vi "MANUALGCODE.vi"(8 "error in (no error)":errorcluster, 9 "PARA":cluster{"STEP":i16, "FEEDRATE":dbl} {"STEP" min=0 max=90 step=2 format="%-1.0f"}, 10 "STATE\nSTAT":enum16{"X-", "X+", "Y-", "Y+", "Z-", "Z+"}(ring), 11 "QUEUE IN":refnum<queue>) -> (0 "error out":errorcluster)   [LabVIEW 2017]
panel:
  out "concatenated string":string
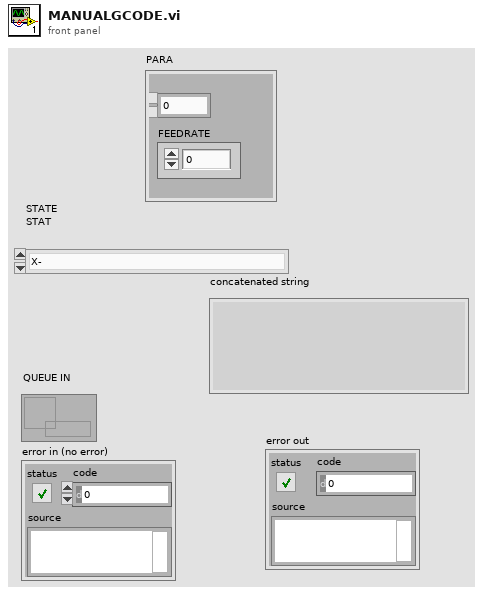
[diagram p1: front panel]
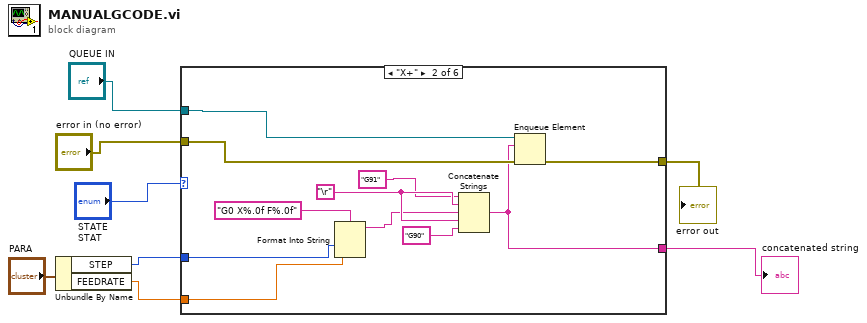
[diagram p0: block diagram]
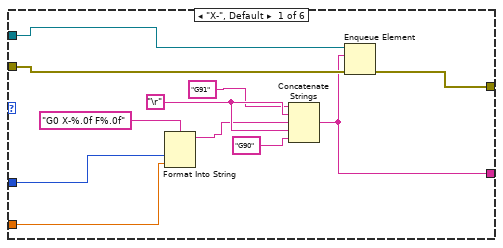
[diagram p2: hidden frame]
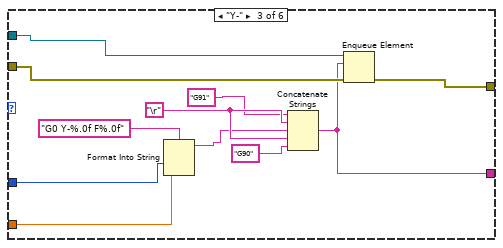
[diagram p3: hidden frame]
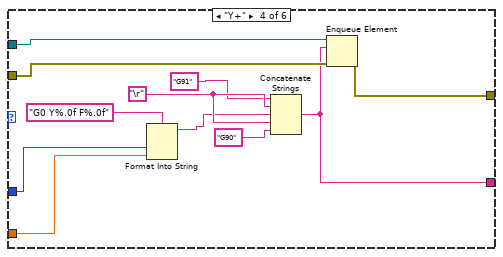
[diagram p4: hidden frame]
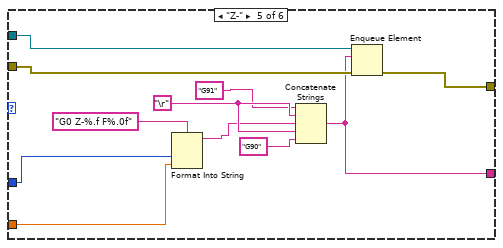
[diagram p5: hidden frame]
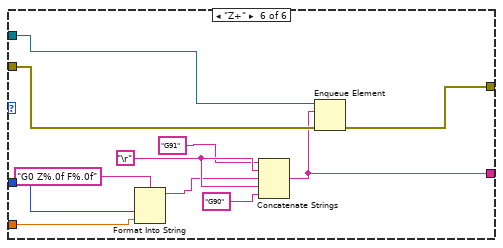
[diagram p6: hidden frame]
diagram:
  n1 = Unbundle By Name("PARA") -> ("STEP"=w1:i16, "FEEDRATE"=w2:dbl)
  n2 = case shown="\"X+\"" "STATE\nSTAT" {
    tunnel: "QUEUE IN" -> [w13 w27 w35 w47 w58 w68]
    tunnel: "error in (no error)" -> [w12 w26 w34 w46 w57 w67]
    tunnel: [w14 w25 w36 w45 w56 w69] -> w5
    tunnel: w2 -> [w10 w20 w31 w43 w54 w65]
    tunnel: [w11 w22 w33 w44 w55 w66] -> w4
    tunnel: w1 -> [w9 w21 w32 w42 w53 w64]
    frame "X-", Default {
      w19 = "\r"
      n3 = Format Into String(format string="G0 X-%.0f F%.0f", w9, w10) -> (resulting string=w15:string)  [unwired: 2 in, 1 out]
      n4 = Concatenate Strings("G91" ("string"), w19, w15, w19, "G90" ("string")) -> (w11:string)
      n5 = Enqueue Element(queue=w13, element=w11, error in (no error)=w12) -> (error out=w14:errorcluster)  [unwired: 1 in, 2 out]
    }
    frame "X+" {
      w30 = "\r"
      n6 = Format Into String(format string="G0 X%.0f F%.0f", w21, w20) -> (resulting string=w23:string)  [unwired: 2 in, 1 out]
      n7 = Concatenate Strings("G91" ("string"), w30, w23, w30, "G90" ("string")) -> (w22:string)
      n8 = Enqueue Element(queue=w27, element=w22, error in (no error)=w26) -> (error out=w25:errorcluster)  [unwired: 1 in, 2 out]
    }
    frame "Y-" {
      w41 = "\r"
      n9 = Format Into String(format string="G0 Y-%.0f F%.0f", w32, w31) -> (resulting string=w37:string)  [unwired: 2 in, 1 out]
      n10 = Concatenate Strings("G91" ("string"), w41, w37, w41, "G90" ("string")) -> (w33:string)
      n11 = Enqueue Element(queue=w35, element=w33, error in (no error)=w34) -> (error out=w36:errorcluster)  [unwired: 1 in, 2 out]
    }
    frame "Y+" {
      w52 = "\r"
      n12 = Format Into String(format string="G0 Y%.0f F%.0f", w42, w43) -> (resulting string=w48:string)  [unwired: 2 in, 1 out]
      n13 = Concatenate Strings("G91" ("string"), w52, w48, w52, "G90" ("string")) -> (w44:string)
      n14 = Enqueue Element(queue=w47, element=w44, error in (no error)=w46) -> (error out=w45:errorcluster)  [unwired: 1 in, 2 out]
    }
    frame "Z-" {
      w63 = "\r"
      n15 = Format Into String(format string="G0 Z-%.f F%.0f", w53, w54) -> (resulting string=w59:string)  [unwired: 2 in, 1 out]
      n16 = Concatenate Strings("G91" ("string"), w63, w59, w63, "G90" ("string")) -> (w55:string)
      n17 = Enqueue Element(queue=w58, element=w55, error in (no error)=w57) -> (error out=w56:errorcluster)  [unwired: 1 in, 2 out]
    }
    frame "Z+" {
      w74 = "\r"
      n18 = Format Into String(format string="G0 Z%.0f F%.0f", w64, w65) -> (resulting string=w70:string)  [unwired: 2 in, 1 out]
      n19 = Concatenate Strings("G91" ("string"), w74, w70, w74, "G90" ("string")) -> (w66:string)
      n20 = Enqueue Element(queue=w68, element=w66, error in (no error)=w67) -> (error out=w69:errorcluster)  [unwired: 1 in, 2 out]
    }
  }
  "error out" <- w5
  "concatenated string" <- w4
